vi "ACT_Loop_n.vi"(0 "SIClass in":refnum<class "SIClass.lvclass">, 5 "Loop ID":enum16{"10", "20", "30", "40"}(ring), 7 "3 JECxx CT001A XQ01":dbl, 9 "3 JECxx CT001B XQ01":dbl, 11 "error in (no error)":errorcluster) -> (8 "Numeric":dbl)   [LabVIEW 2022 SP3, in "SIClass.lvclass"]
uses:
  SI101/SI101_AverageReactorCoolantTemperature.lvclass/SI101_AverageReactorCoolantTemperature.ctl
  SIClass.lvclass
  SIClass.lvclass/SIClass.ctl
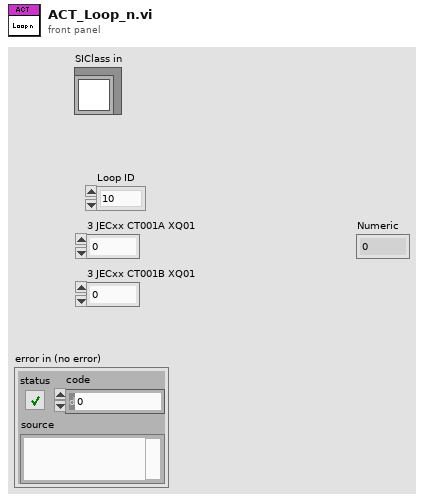
[diagram p1: front panel]
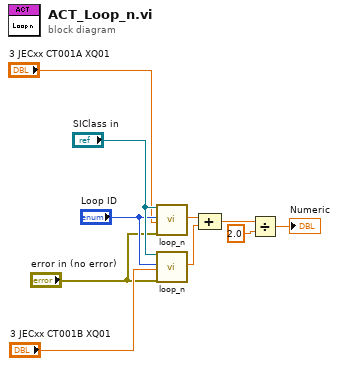
[diagram p0: block diagram]
diagram:
  n1 = call-dynamic "loop_n.vi"("SIClass in"="SIClass in", "Loop ID"="Loop ID", "Input"="3 JECxx CT001A XQ01", "error in (no error)"="error in (no error)") -> ("Output"=w4:dbl)  [unwired: 13 in, 2 out]
  n2 = call-dynamic "loop_n.vi"("SIClass in"="SIClass in", "Loop ID"="Loop ID", "Input"="3 JECxx CT001B XQ01", "error in (no error)"="error in (no error)") -> ("Output"=w5:dbl)  [unwired: 13 in, 2 out]
  n3 = Compound Arithmetic op=ADD(w4, w5) -> (w6:dbl)
  n4 = Divide(x=w6, y=2.0) -> (x/y=→"Numeric":dbl)
